vi "Push_Data_Client.vi"(5 "Archive File?":bool, 6 "application reference":refnum<vi>, 7 "error in (no error)":errorcluster, 9 "File Path relative to Sync Folder":path=path "/Lacie_20/test", 10 "Path of Folder relative to EnFlo_Data Root":path) -> (0 "error out":errorcluster)   [LabVIEW 2011]
uses:
  Anemometry/Anemometry Sub Vis/Globals/Constants_global.vi
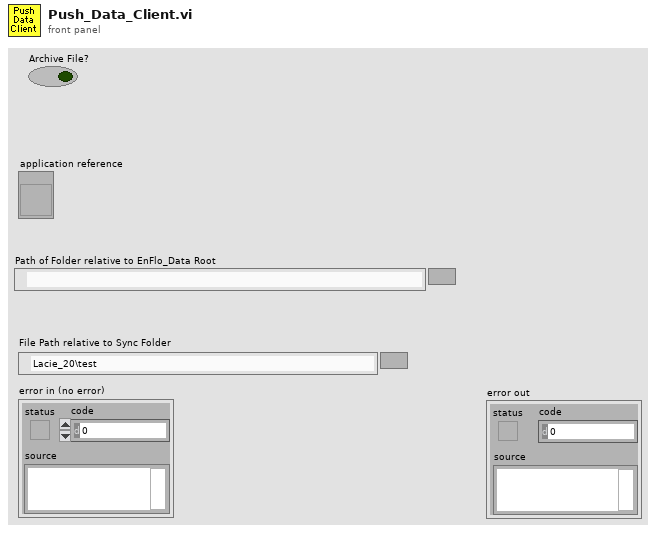
[diagram p1: front panel]
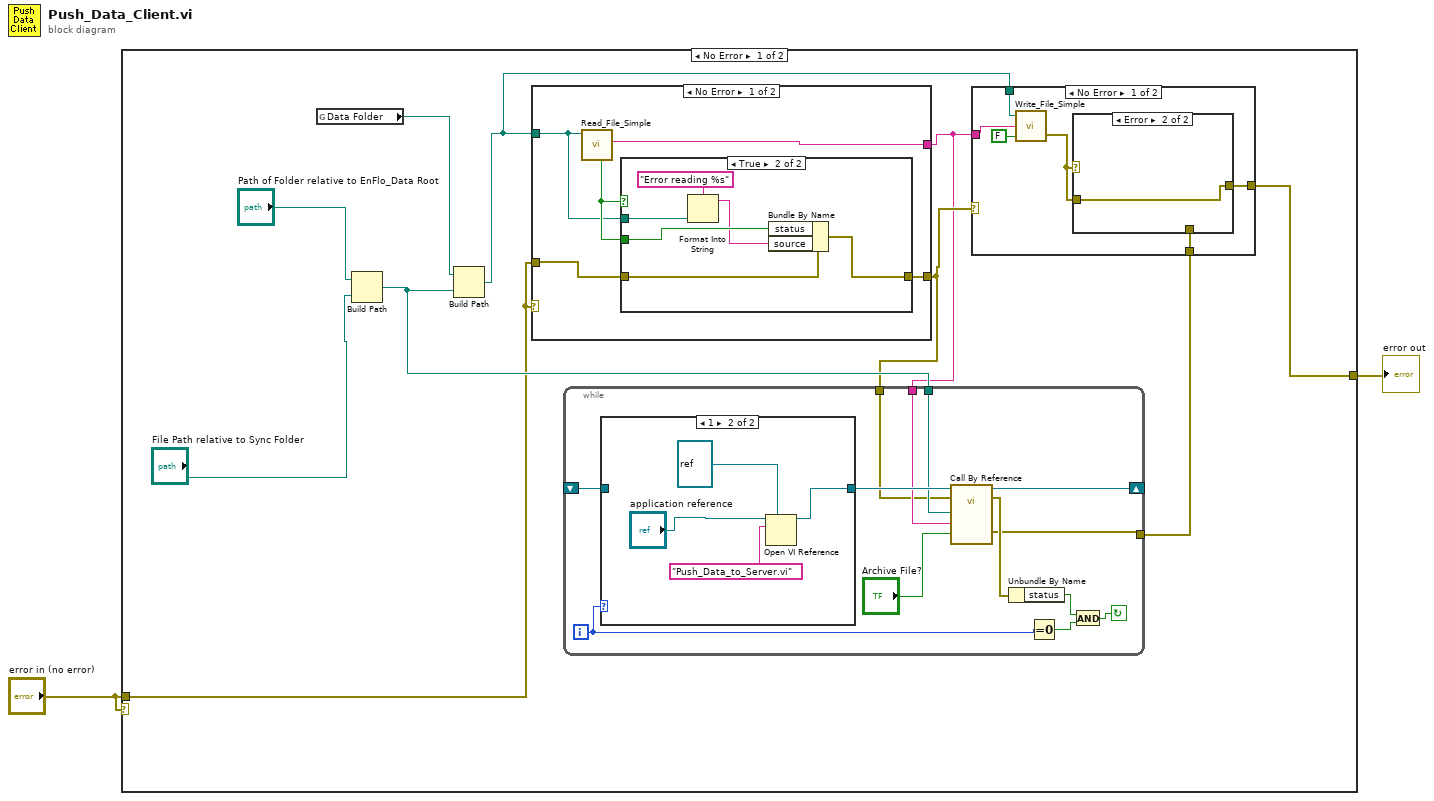
[diagram p0: block diagram]
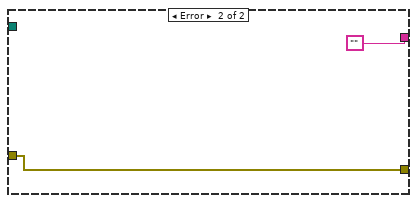
[diagram p5: hidden frame]
diagram:
  n1 = case shown="No Error" "error in (no error)" {
    tunnel: [w4 w54] -> w2
    tunnel: "error in (no error)" -> [w8 w54]
    frame No Error {
      n2 = global read "Constants_global.vi" "Data Folder"() -> (w9:path)
      n3 = Build Path(base path="Path of Folder relative to EnFlo_Data Root", name or relative path="File Path relative to Sync Folder") -> (appended path=w10:path)
      n4 = Build Path(base path=w9, name or relative path=w10) -> (appended path=w7:path)
      n5 = case shown="No Error" w8 {
        tunnel: w7 -> [w24 _]
        tunnel: [w26 ""] -> w5
        tunnel: [w23 w34] -> w6
        tunnel: w8 -> [w22 w34]
        frame No Error {
          n6 = call "Read_File_Simple.vi"("Filename"=w24) -> ("Error?"=w25:bool, "string"=w26:string)  [unwired: 4 in, 4 out]
          n7 = case shown="True" w25 {
            tunnel: w22 -> [w27 w33]
            tunnel: w25 -> [_ w32]
            tunnel: w24 -> [_ w30]
            tunnel: [w27 w28] -> w23
            frame False {
            }
            frame True {
              n8 = Format Into String(format string="Error reading %s", w30) -> (resulting string=w29:string)  [unwired: 2 in, 1 out]
              n9 = Bundle By Name(cluster=w33, "status"=w32, "source"=w29) -> (w28:errorcluster)
            }
          }
        }
        frame Error {
        }
      }
      n10 = while {
        shift-right: [w46] -> _
        shift-left: _ -> [w48]
        tunnel: w10 -> [w41]
        tunnel: w5 -> [w40]
        tunnel: [w38] -> w3
        tunnel: w6 -> [w36]
        i -> [w45]
        stop <- w42 continue-if-true
        n11 = case shown="1" w45 {
          tunnel: w48 -> [w49 _]
          tunnel: [w49 w53] -> w47
          frame 0, Default {
          }
          frame 1 {
            n12 = Open VI Reference(type specifier VI Refnum (for type only)=refnum<vi> refnum ("Push Data Server"), application reference (local)="application reference", vi path="Push_Data_to_Server.vi") -> (vi reference=w53:refnum<vi>)  [unwired: 1 in, 3 out]
          }
        }
        n13 = call-by-ref "?"(reference=w47, error in=w36, "Archive File?"="Archive File?", "Zip String"=w40, "Relative Path"=w41) -> (reference out=w46:refnum<vi>, error out=w39:errorcluster, "error out"=w38:errorcluster)  [unwired: 1 in]
        n14 = Unbundle By Name(w39) -> ("status"=w43:bool)
        n15 = Equal To 0?(x=w45) -> (x = 0?=w44:bool)
        n16 = And(x=w43, y=w44) -> (x .and. y?=w42:bool)
      }
      n17 = case shown="No Error" w6 {
        tunnel: w5 -> [w17 _]
        tunnel: w7 -> [w18 _]
        tunnel: [w15 w21] -> w4
        tunnel: w3 -> [w14 w21]
        frame No Error {
          n18 = call "Write_File_Simple.vi"("append to file? (new file:F)"=FALSE, "character string"=w17, "file path"=w18) -> ("error out"=w13:errorcluster)  [unwired: 1 out]
          n19 = case shown="Error" w13 {
            tunnel: [w19 w20] -> w15
            tunnel: w14 -> [w19 _]
            tunnel: w13 -> [_ w20]
            frame No Error {
            }
            frame Error {
            }
          }
        }
        frame Error {
        }
      }
    }
    frame Error {
    }
  }
  "error out" <- w2
